vi "SCCAPI Configure Project.vi"(8 "error in (no error)":errorcluster, 9 "configuration data in":string) -> (0 "error out":errorcluster, 1 "configuration data out":string, 2 "status message":string, 5 "dialog box cancelled?":bool)   [LabVIEW 2017, in "NI_SCC.lvlib"]
uses:
  <vilib>/SourceControl/sccapi/NI_SCC.lvlib
  <vilib>/SourceControl/sccapi/SCCAPI SCC Operations.ctl
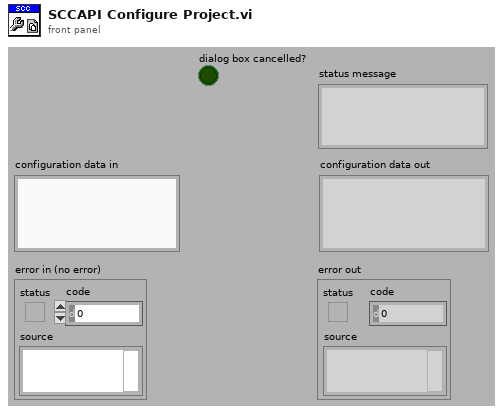
[diagram p1: front panel]
types:
  T1 = typedef "NI_SCC.lvlib/SCCAPI SCC Operations.ctl" = enum16{"Add", "Check In", "Check Out", "Close Project", "Compare Files", "Compare VIs", "Configure Project", "File History", "File Properties", "File Status", "Find All Providers", "Get Advanced Command Options", "Get File Copy", "Get Latest Version", "Get Project Name", "Get StaticVI Path", "Initialize", "Not A Source Control Reference", "Open Project", "Provider Supports Functionality", "Remove", "Run Provider", "Undo Check Out", "Uninitialize", "Is File In Local Path"}
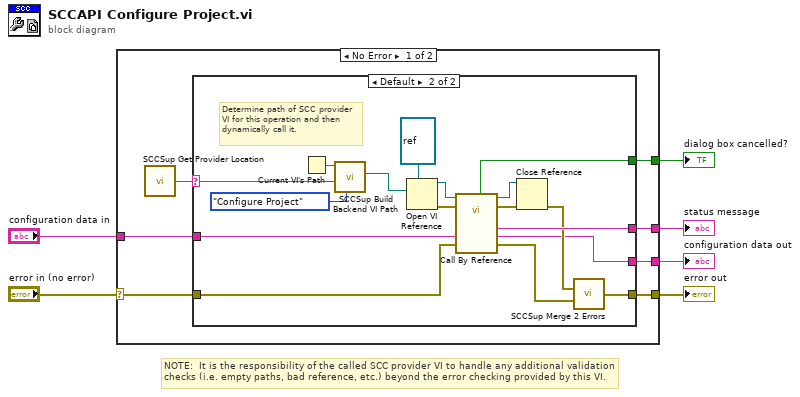
[diagram p0: block diagram]
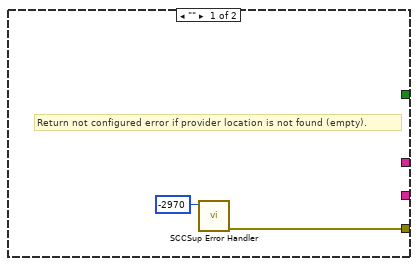
[diagram p2: hidden frame]
diagram:
  # "NOTE:  It is the responsibility of the called SCC provider VI to handle any additional validation checks (i.e. empty paths, bad reference, etc.) beyond the error checking provided by this VI."
  n1 = case shown="No Error" "error in (no error)" {
    selector: "error in (no error)" -> [w10 w33]
    tunnel: [w13 w33] -> w5
    tunnel: [w12 _] -> w4
    tunnel: [w9 _] -> w3
    tunnel: "configuration data in" -> [w8 _]
    tunnel: [w7 _] -> w1
    frame No Error {
      n2 = call <vilib>:"SCCSup Get Provider Location.vi"() -> ("provider location"=w11:string)  [unwired: 6 in]
      n3 = case shown="Default" w11 {
        selector: w11 -> [_ w21]
        tunnel: [w14 w32] -> w13
        tunnel: [_ w26] -> w12
        tunnel: w10 -> [_ w20]
        tunnel: [_ w19] -> w9
        tunnel: w8 -> [_ w18]
        tunnel: [_ w16] -> w7
        frame "" {
          # "Return not configured error if provider location is not found (empty)."
          n4 = call <vilib>:"SCCSup Error Handler.vi"("scc error code"=-2970 ("code")) -> ("error out"=w14:errorcluster)  [unwired: 10 in]
        }
        frame Default {
          # "Determine path of SCC provider VI for this operation and then dynamically call it."
          n5 = Current VI's Path() -> (path=w22:path)
          n6 = call <vilib>:"SCCSup Build Backend VI Path.vi"("scc operation"=SCCAPI_SCC_Operations."Configure Project", "provider location"=w21, "caller path"=w22) -> ("scc backend VI path"=w24:path)  [unwired: 8 in]
          n7 = Open VI Reference(type specifier VI Refnum (for type only)=refnum<vi> refnum, vi path=w24) -> (vi reference=w30:refnum<vi>, error out=w29:errorcluster)  [unwired: 4 in]
          n8 = call-by-ref "?"(reference=w30, error in=w29, "error in (no error)"=w20, "configuration data in"=w18) -> (reference out=w28:refnum<vi>, error out=w27:errorcluster, 0:"error out"=w17:errorcluster, "configuration data out"=w16:string, "status message"=w26:string, "dialog box cancelled?"=w19:bool)  [unwired: 6 in]
          n9 = Close Reference(reference=w28, error in (no error)=w27) -> (error out=w25:errorcluster)
          n10 = call <vilib>:"SCCSup Merge 2 Errors.vi"("Error IO 1"=w25, "Error IO 2"=w17) -> ("Error IO out"=w32:errorcluster)  [unwired: 13 in]
        }
      }
    }
    frame Error {
    }
  }
  "error out" <- w5
  "status message" <- w4
  "dialog box cancelled?" <- w3
  "configuration data out" <- w1
